vi "RichToFlatcif_plugincore_GetConfigResponse.vi"(5 "OutputClusterType":T1, 11 "InputCluster":T3) -> (3 "OutputCluster":T1)   [LabVIEW 2021, in "CIFCorePlugin_server.lvlib"]
uses:
  CIFCorePlugin_server.lvlib
  cif_plugincore_GetConfigResponse.ctl
  cif_plugincore_Configuration.ctl
  cif_plugincore_GetConfigResponse_Flat.ctl
  cif_plugincore_Configuration_Flat.ctl
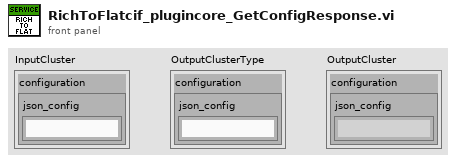
[diagram p1: front panel]
types:
  T1 = typedef "CIFCorePlugin_server.lvlib/cif_plugincore_GetConfigResponse_Flat.ctl" = cluster{"configuration":T2}
  T2 = typedef "CIFCorePlugin_server.lvlib/cif_plugincore_Configuration_Flat.ctl" = cluster{"json_config":string}
  T3 = typedef "CIFCorePlugin_server.lvlib/cif_plugincore_GetConfigResponse.ctl" = cluster{"configuration":T4}
  T4 = typedef "CIFCorePlugin_server.lvlib/cif_plugincore_Configuration.ctl" = cluster{"json_config":string}
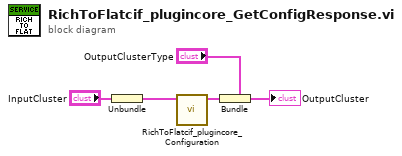
[diagram p0: block diagram]
diagram:
  n1 = Unbundle "Unbundle"("InputCluster") -> ("configuration"=w2:T4)
  n2 = call "RichToFlatcif_plugincore_Configuration.vi"("InputCluster"=w2) -> ("OutputCluster"=w1:T2)  [unwired: 10 in]
  n3 = Bundle "Bundle"(cluster="OutputClusterType", "configuration"=w1) -> (→"OutputCluster":T1)
